vi "Initialize.vi"(8 "error in (no error)":errorcluster, 10 "Settings":variant, 11 "Modbus PLC in":refnum<class "Modbus PLC.lvclass">) -> (0 "error out":errorcluster, 3 "Modbus PLC out":refnum<class "Modbus PLC.lvclass">)   [LabVIEW 2023, in "Modbus PLC.lvlib" / "Modbus PLC.lvclass"]
uses:
  Modbus PLC.lvclass
  Settings.ctl
  Modbus PLC.lvclass/Modbus PLC.ctl
  <vilib>/NI/Modbus Library/API/Wrapper/Create TCP Master.vi
  Workers Hardware/Workers/Base Classes/Base Hardware/Base Hardware.lvclass
  <vilib>/NI/Modbus Library/API/Wrapper/API Main.lvlib
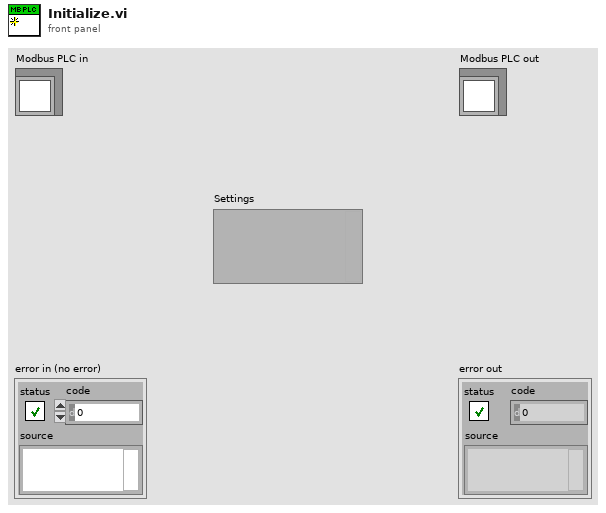
[diagram p1: front panel]
types:
  T1 = typedef "Modbus PLC.lvlib/Modbus PLC.lvclass/Settings.ctl" = cluster{"IP Address":string, "Port":u16}
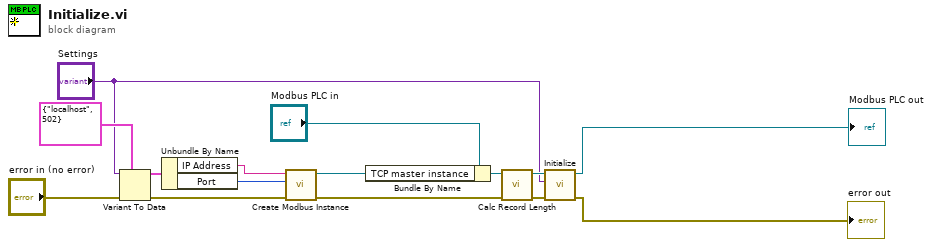
[diagram p0: block diagram]
diagram:
  n1 = Variant To Data(error in="error in (no error)", type=T1 {"IP Address"="localhost", "Port"=502} ("Settings"), Variant="Settings") -> (data=w13:T1, error out=w5:errorcluster)
  n2 = Unbundle By Name(w13) -> ("IP Address"=w7:string, "Port"=w6:u16)
  n3 = call-poly <vilib>:"Create Modbus Instance.vi"("error in"=w5, "port (502)"=w6, "address"=w7) -> ("error out"=w4:errorcluster, "TCP master instance"=w3:refnum<class "Modbus Master.lvclass">)  [unwired: 7 in]
  n4 = Bundle By Name(cluster="Modbus PLC in", "TCP master instance"=w3) -> (w11:refnum<class "Modbus PLC.lvclass">)
  n5 = call "Calc Record Length.vi"("error in (no error)"=w4, "Modbus PLC in"=w11) -> ("error out"=w10:errorcluster, "Modbus PLC out"=w9:refnum<class "Modbus PLC.lvclass">)  [unwired: 8 in]
  n6 = call-parent "Initialize.vi"("error in (no error)"=w10, "Settings"="Settings", "Base Hardware in"=w9) -> ("error out"=→"error out":errorcluster, "Base Hardware out"=→"Modbus PLC out":refnum<class "Modbus PLC.lvclass">)  [unwired: 7 in]
